vi "Find first nonzero element in array.vi"(8 "error in (no error)":errorcluster, 11 "Array in":i16[](array[numeric])) -> (0 "error out":errorcluster, 1 "found?":bool, 2 "Element":i16, 3 "Index":i32)   [LabVIEW 2012]
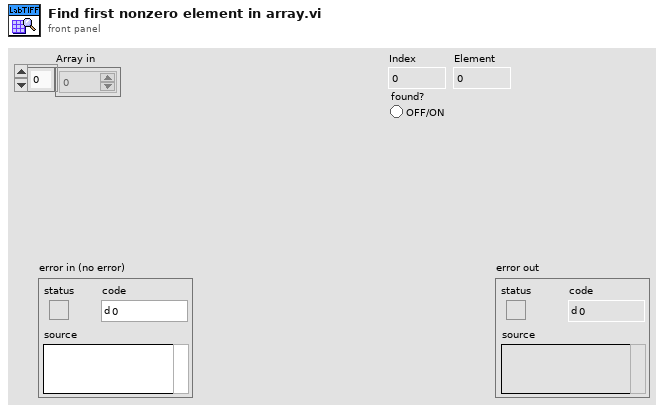
[diagram p1: front panel]
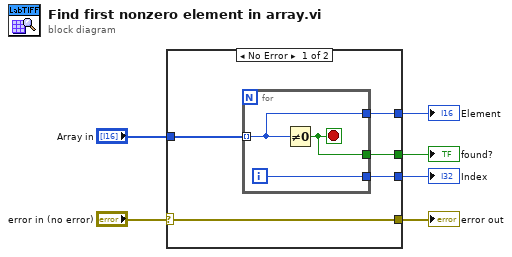
[diagram p0: block diagram]
diagram:
  n1 = case shown="No Error" "error in (no error)" {
    selector: "error in (no error)" -> [w11 w15]
    tunnel: [w11 w15] -> w5
    tunnel: "Array in" -> [w10 _]
    tunnel: [w9 _] -> w3
    tunnel: [w8 _] -> w1
    tunnel: [w7 _] -> w2
    frame No Error {
      n2 = for {
        tunnel: w10 -> [w13] mode=indexing
        tunnel: [w14] -> w9
        tunnel: [w13] -> w8
        tunnel: [w12] -> w7
        i -> [w14]
        stop <- w12 stop-if-true
        n3 = Not Equal To 0?(x=w13) -> (x != 0?=w12:bool)
      }
    }
    frame Error {
    }
  }
  "error out" <- w5
  "Index" <- w3
  "found?" <- w2
  "Element" <- w1
